vi "AlliGator Add Python Functions to Object Menu.vi"(8 "error in (no error)":errorcluster, 10 "Menu in":refnum<k9>, 11 "Object Refnum":refnum<vi>) -> (0 "error out":errorcluster, 2 "Menu out":refnum<k9>, 3 "Object Refnum dup":refnum<vi>)   [LabVIEW 2021, in "AlliGator Python Plugins.lvlib"]
doc: "Adds python function to object menu."
uses:
  AlliGator Python Plugins.lvlib
panel:
  # "see the AlliGator License on the block diagram (Ctrl+E or Window:Show Block Diagram)"
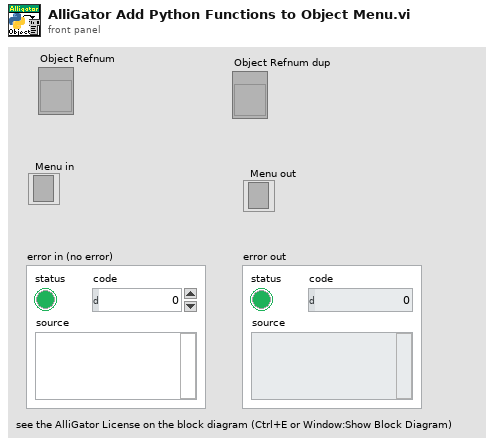
[diagram p1: front panel]
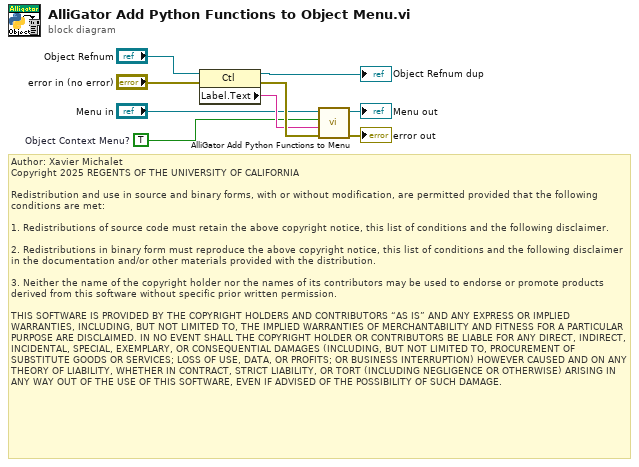
[diagram p0: block diagram]
diagram:
  w1 = TRUE  # Object Context Menu?
  # "Author: Xavier Michalet\nCopyright 2025 REGENTS OF THE UNIVERSITY OF CALIFORNIA\n\nRedistribution and use in source and binary forms, with or without modification, are permitted provided that the following conditions are met:\n\n1. Redistributions of source code must retain the above copyright notice, this list of conditions and the following disclaimer.\n\n2. Redistributions in binary form must reproduce the above copyright notice, this list of conditions and the following disclaimer in the documentation and/or other materials provided with the distribution.\n\n3. Neither the name of the copyright holder nor the names of its contributors may be used to endorse or promote products derived from this software without specific prior written permission.\n\nTHIS SOFTWARE IS PROVIDED BY THE COPYRIGHT HOLDERS AND CONTRIBUTORS “AS IS” AND ANY EXPRESS OR IMPLIED WARRANTIES, INCLUDING, BUT NOT LIMITED TO, THE IMPLIED WARRANTIES OF MERCHANTABILITY AND FITNESS FOR A PARTICULAR PURPOSE ARE DISCLAIMED. IN NO EVENT SHALL THE COPYRIGHT HOLDER OR CONTRIBUTORS BE LIABLE FOR ANY DIRECT, INDIRECT, INCIDENTAL, SPECIAL, EXEMPLARY, OR CONSEQUENTIAL DAMAGES (INCLUDING, BUT NOT LIMITED TO, PROCUREMENT OF SUBSTITUTE GOODS OR SERVICES; LOSS OF USE, DATA, OR PROFITS; OR BUSINESS INTERRUPTION) HOWEVER CAUSED AND ON ANY THEORY OF LIABILITY, WHETHER IN CONTRACT, STRICT LIABILITY, OR TORT (INCLUDING NEGLIGENCE OR OTHERWISE) ARISING IN ANY WAY OUT OF THE USE OF THIS SOFTWARE, EVEN IF ADVISED OF THE POSSIBILITY OF SUCH DAMAGE."
  n1 = property class="Ctl"(reference="Object Refnum", error in="error in (no error)") -> (reference out=→"Object Refnum dup":refnum<vi>, error out=w9:errorcluster, "Label.Text"=w7:string)
  n2 = call "AlliGator Add Python Functions to Menu.vi"("error in (no error)"=w9, "Parent Menu Tag"=w7, "Object Context Menu?"=w1, "Menu in"="Menu in") -> ("error out"=→"error out":errorcluster, "Menu out"=→"Menu out":refnum<k9>)  [unwired: 6 in]
